vi "Config Dev Average.vi"(8 "error in":errorcluster, 10 "Average Time (0.1 sec)":dbl=0.1 min=0.0 max=999999.9, 11 "VISA resource name":refnum<visa-resource-name>) -> (0 "error out":errorcluster, 3 "VISA resource name out":refnum<visa-resource-name>)   [LabVIEW 2018, in "Andeen-Hagerling 2700.lvlib"]
doc: "This VI sets the minimum time interval during which measurement samples are averaged in the deviation N Data Stream case or during which the occurrence of an error is watched for in the deviation E Data Stream case."
uses:
  Andeen-Hagerling 2700.lvlib
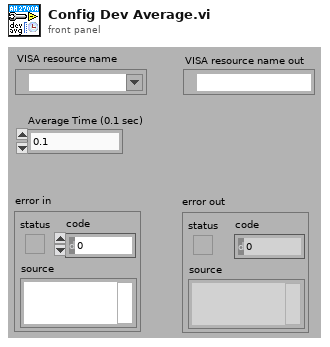
[diagram p1: front panel]
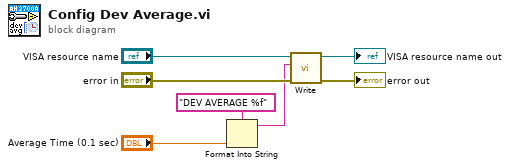
[diagram p0: block diagram]
diagram:
  n1 = Format Into String(format string="DEV AVERAGE %f", "Average Time (0.1 sec)") -> (resulting string=w2:string)  [unwired: 2 in, 1 out]
  n2 = call "Write.vi"("error in"="error in", "command"=w2, "VISA resource name"="VISA resource name") -> ("error out"=→"error out":errorcluster, "VISA resource name out"=→"VISA resource name out":refnum<visa-resource-name>)  [unwired: 7 in]
